vi "matrix-AVG.vi"() -> ()   [LabVIEW 2018]
doc: "Average Matrix\n\n\nAndré Romero - 2022\nandretec@ifsc.usp.br"
panel:
  out "output Matrix":dbl[][](array[numeric])
  in  "input Matrix":dbl[][][](array[numeric])
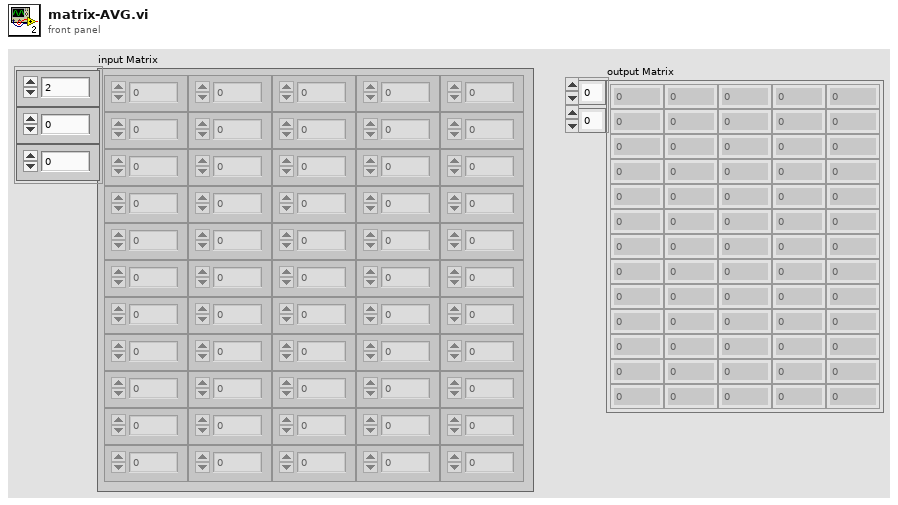
[diagram p1: front panel]
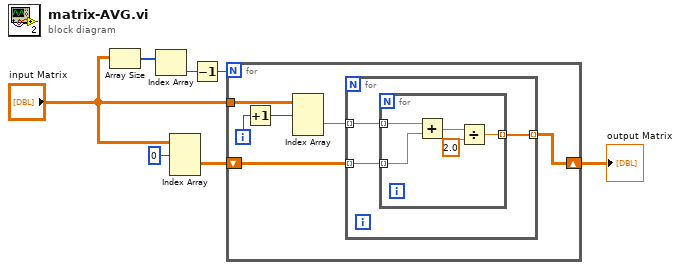
[diagram p0: block diagram]
diagram:
  n1 = Array Size(array="input Matrix") -> (size(s)=w7:i32[])
  n2 = Index Array(array=w7) -> (element=w6:i32)  [unwired: 1 in]
  n3 = Index Array(array="input Matrix", index (dim 0)=0 ("index (page)")) -> (element=w1:dbl[][])  [unwired: 2 in]
  n4 = Decrement(x=w6) -> (x-1=w4:i32)
  n5 = for {
    N: w4 -> [_]
    tunnel: "input Matrix" -> [w12]
    shift-right: [w9] -> w5
    shift-left: w1 -> [w11]
    i -> [w13]
    n6 = Increment(x=w13) -> (x+1=w8:i32)
    n7 = Index Array(array=w12, index (dim 0)=w8) -> (element=w10:dbl[][])  [unwired: 2 in]
    n8 = for {
      tunnel: w11 -> [w16] mode=indexing
      tunnel: w10 -> [w15] mode=indexing
      tunnel: [w14] -> w9 mode=indexing
      n9 = for {
        tunnel: w16 -> [w20] mode=indexing
        tunnel: w15 -> [w21] mode=indexing
        tunnel: [w17] -> w14 mode=indexing
        n10 = Add(x=w21, y=w20) -> (x+y=w19:dbl)
        n11 = Divide(x=w19, y=2.0) -> (x/y=w17:dbl)
      }
    }
  }
  "output Matrix" <- w5
